vi "Plot XY.vi"(8 "error in (no error)":errorcluster, 10 "Channel":u8, 11 "Micron Optics Recorder in":refnum<class "Ruby Spectra.lvclass">) -> (0 "error out":errorcluster, 3 "Micron Optics Recorder out":refnum<class "Ruby Spectra.lvclass">)   [LabVIEW 2024, in "Ruby Spectra.lvclass"]
uses:
  Ruby Spectra.lvclass
  Spectrometer/Spectrometer.lvclass
  Ruby Spectra.lvclass/Ruby Spectra.ctl
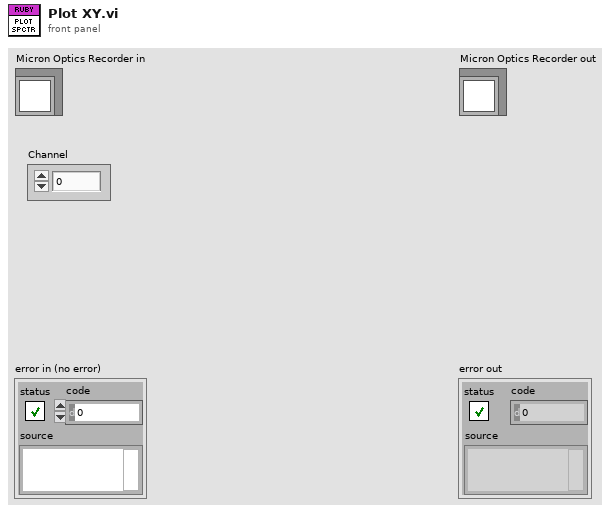
[diagram p1: front panel]
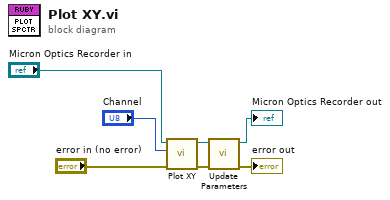
[diagram p0: block diagram]
diagram:
  n1 = call-parent "Plot XY.vi"("error in (no error)"="error in (no error)", "Channel"="Channel", "Micron Optics Recorder in"="Micron Optics Recorder in") -> ("error out"=w7:errorcluster, "Micron Optics Recorder out"=w2:refnum<class "Ruby Spectra.lvclass">)  [unwired: 7 in]
  n2 = call-dynamic "Update Parameters.vi"("error in (no error)"=w7, "Ruby Spectra in"=w2) -> ("error out"=→"error out":errorcluster, "Ruby Spectra out"=→"Micron Optics Recorder out":refnum<class "Ruby Spectra.lvclass">)  [unwired: 8 in]
